vi "Tx Parser.vi"(8 "Error In":errorcluster, 11 "Data In":T2={"Console log"="", "Application directory"=path "", "GUI_Events"={"To_GUI-Producer"=refnum, "To_GUI-Error_message"=refnum, "To_GUI-msg_list"=refnum, "To_GUI-Session"=refnum, "To_GUI-Pre-Session"=refnum, "To_GUI-Consumer"=refnum}, "Function_Queue"={"Queue_MIDI_Handler"=refnum, "Queue_Session"=refnum, "Queue_Producer"=refnum, "Queue_Consumer"=refnum}, "Timout-Time[ms]"=0, "MIDI-Messages"=[], "Selected Consumer"=enum."Random", "Com Session State"=enum."Active Session", "Result Data"={"Diff"=[], "Tx Byte"=[], "Rx Byte"=[], "Send Log"=[]}, "Get #"=[], "CPU(ms)"=0}) -> (0 "Error Out":errorcluster, 3 "Data Out":T2={"Console log"="", "Application directory"=path "", "GUI_Events"={"To_GUI-Producer"=refnum, "To_GUI-Error_message"=refnum, "To_GUI-msg_list"=refnum, "To_GUI-Session"=refnum, "To_GUI-Pre-Session"=refnum, "To_GUI-Consumer"=refnum}, "Function_Queue"={"Queue_MIDI_Handler"=refnum, "Queue_Session"=refnum, "Queue_Producer"=refnum, "Queue_Consumer"=refnum}, "Timout-Time[ms]"=0, "MIDI-Messages"=[], "Selected Consumer"=enum."Random", "Com Session State"=enum."Active Session", "Result Data"={"Diff"=[], "Tx Byte"=[], "Rx Byte"=[], "Send Log"=[]}, "Get #"=[], "CPU(ms)"=0})   [LabVIEW 2019]
doc: "This VI is used as a standard template for subVI's."
uses:
  Common/Controls/Application_Data.ctl
  Common/Controls/App_Events.ctl
  Common/Controls/App_Queues.ctl
  Common/Controls/Application_Message.ctl
  Common/Controls/Application_State.ctl
  Controls/MIDI-Message_Array.ctl
  Controls/MIDI-Message_Cluster.ctl
  Controls/Meta_Commands.ctl
  Consumer/Controls/Consumer_States.ctl
  Producer/Controls/Session_State.ctl
  Consumer/Controls/Consumer_Result.ctl
  <vilib>/Utility/error.llb/DialogType.ctl
panel:
  in  "Control Tab":T1(tab)
  out "Console Out":string
  out "Error Message":string
  out "VI-filename":string
  out "VI Path":path
  out "Code Size":u32
  out "Revision Number":u32
  in  "Tool Bar:Visible":bool
  in  "Execution:Show Front Panel On Call":bool
  out "VI-Name":string
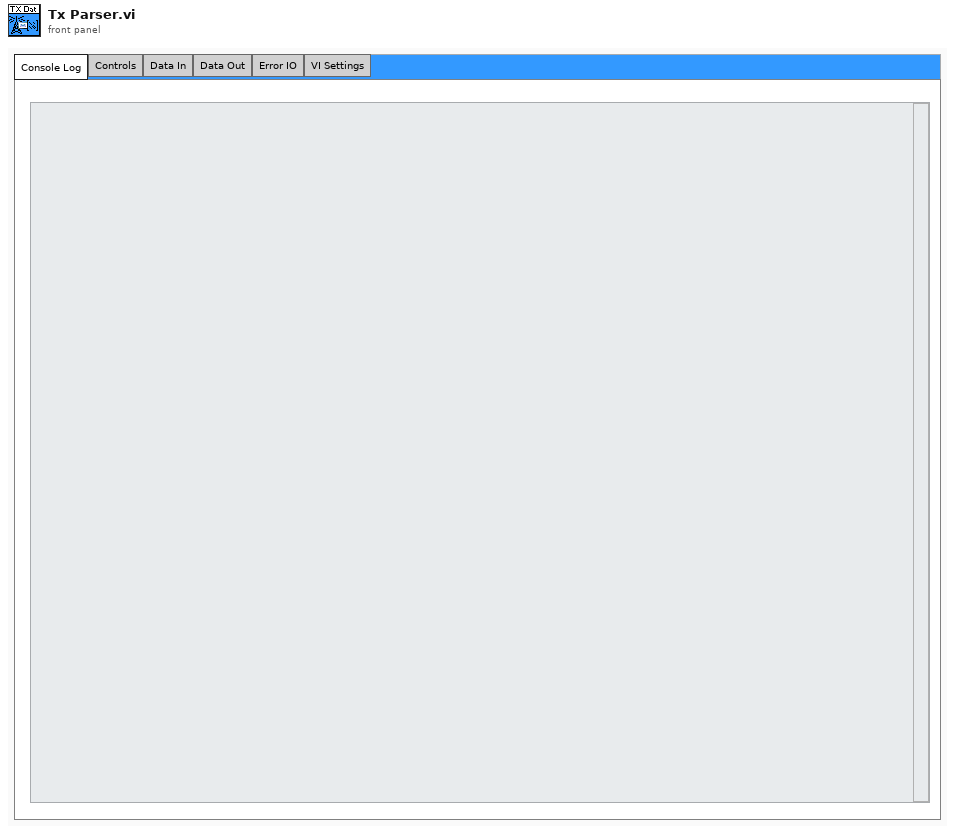
[diagram p1: front panel]
types:
  T1 = enum32{"Console Log", "Controls", "Data In", "Data Out", "Error IO", "VI Settings"}
  T2 = typedef "Application_Data.ctl" = cluster{"Console log":string, "Application directory":path, "GUI_Events":T3, "Function_Queue":T4, "Timout-Time[ms]":i32, "MIDI-Messages":T5, "Selected Consumer":T8, "Com Session State":T9, "Result Data":T10, "Get #":bool[], "CPU(ms)":u32}
  T3 = typedef "App_Events.ctl" = cluster{"To_GUI-Producer":refnum<user-event>, "To_GUI-Error_message":refnum<user-event>, "To_GUI-msg_list":refnum<user-event>, "To_GUI-Session":refnum<user-event>, "To_GUI-Pre-Session":refnum<user-event>, "To_GUI-Consumer":refnum<user-event>}
  T4 = typedef "App_Queues.ctl" = cluster{"Queue_MIDI_Handler":refnum<queue>, "Queue_Session":refnum<queue>, "Queue_Producer":refnum<queue>, "Queue_Consumer":refnum<queue>}
  T5 = typedef "MIDI-Message_Array.ctl" = T6[]
  T6 = typedef "MIDI-Message_Cluster.ctl" = cluster{"Message Name":string, "Meta value":i32, "Datastring":string, "Datatype":T7}
  T7 = typedef "Meta_Commands.ctl" = enum16{"No Data", "Pause", "Loop", "Wait for Rx", "Delay", "Break", "MIDI"}
  T8 = typedef "Consumer_States.ctl" = enum16{"Random", "ECG", "Strech-Patch"}
  T9 = typedef "Session_State.ctl" = enum16{"Wait to begin", "Active Session", "Pause", "Wait for Response", "Stop", "Restart", "Inspect", "Exit"}
  T10 = typedef "Consumer_Result.ctl" = cluster{"Diff":bool[], "Tx Byte":string[], "Rx Byte":string[], "Send Log":string[]}
  T11 = typedef "DialogType.ctl" = u16
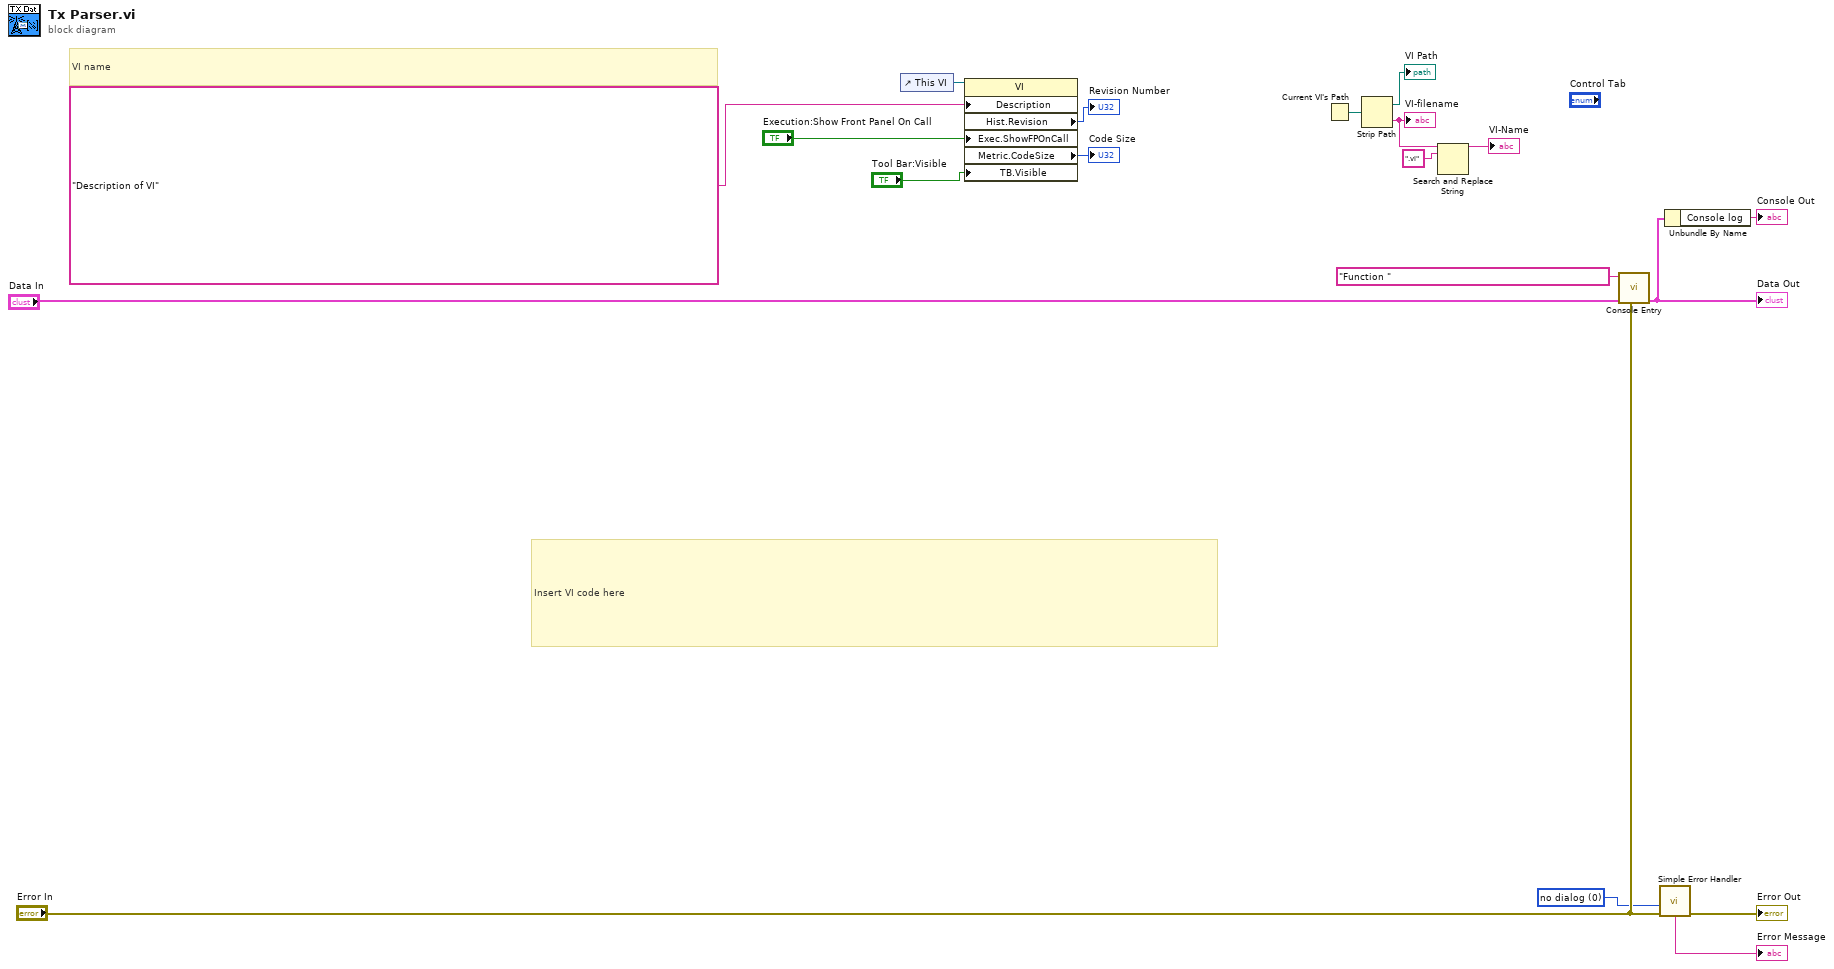
[diagram p0: block diagram]
diagram:
  w1 = T11 0 items=["no dialog", "OK message", "continue or stop message", "OK message + warnings", "continue/stop + warnings"] ("type of dialog (OK msg:1)")
  # "Insert VI code here"
  # "VI name"
  n1 = control-ref of="This VI"() -> (w11:refnum<vi>)
  n2 = property class="VI"(reference=w11, "Description"="Description of VI", "Exec.ShowFPOnCall"="Execution:Show Front Panel On Call", "TB.Visible"="Tool Bar:Visible") -> ("Hist.Revision"=→"Revision Number":u32, "Metric.CodeSize"=→"Code Size":u32)  [unwired: 1 in, 2 out]
  n3 = Current VI's Path() -> (path=w19:path)
  n4 = Strip Path(path=w19) -> (stripped path=→"VI Path":path, name=w8:string)
  "VI-filename" <- w8
  n5 = Search and Replace String(input string=w8, search string=".vi") -> (result string=→"VI-Name":string)  [unwired: 6 in, 3 out]
  n6 = call "Console Entry.vi"("Error In"="Error In", "Data In"="Data In", "Console Entry"="Function ") -> ("Data out"=w6:T2)  [unwired: 8 in]
  "Data Out" <- w6
  n7 = call <vilib>:"Simple Error Handler.vi"("type of dialog (OK msg:1)"=w1, "error in (no error)"="Error In") -> ("error out"=→"Error Out":errorcluster, "message"=→"Error Message":string)  [unwired: 3 in, 3 out]
  n8 = Unbundle By Name(w6) -> ("Console log"=→"Console Out":string)
